vi "Update Core.vi"(8 "error in (no error)":cluster{"状态":bool, "代码":i32, "源":string} caption="错误输入（无错误）", 11 "水位控制器输入":refnum<class "Level Controller.lvclass">) -> (0 "error out":cluster{"状态":bool, "代码":i32, "源":string} caption="错误输出", 3 "水位控制器输出":refnum<class "Level Controller.lvclass">)   [LabVIEW 2015, in "Level Controller.lvlib" / "Level Controller.lvclass"]
doc: "子类绝不可对该VI进行重写。该VI通过“定时循环操作者”父类定义。该水位控制器中，“更新”操作即对水位控制器监控的变量进行检查，然后根据该变量是否高于/低于死区范围执行状态更改。"
uses:
  Level Controller.lvclass
  Level Controller.lvclass/Level Controller.ctl
  Value Position.ctl
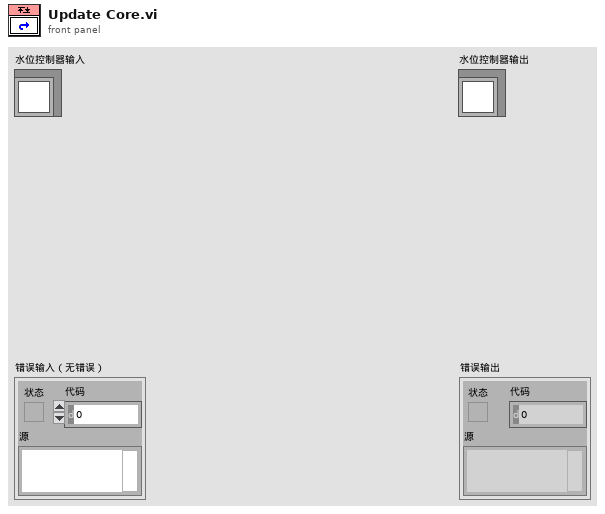
[diagram p1: front panel]
types:
  T1 = typedef "Level Controller.lvlib/Level Controller.lvclass/Value Position.ctl" = enum16{"Never Assigned", "Above Level", "Below Level"}
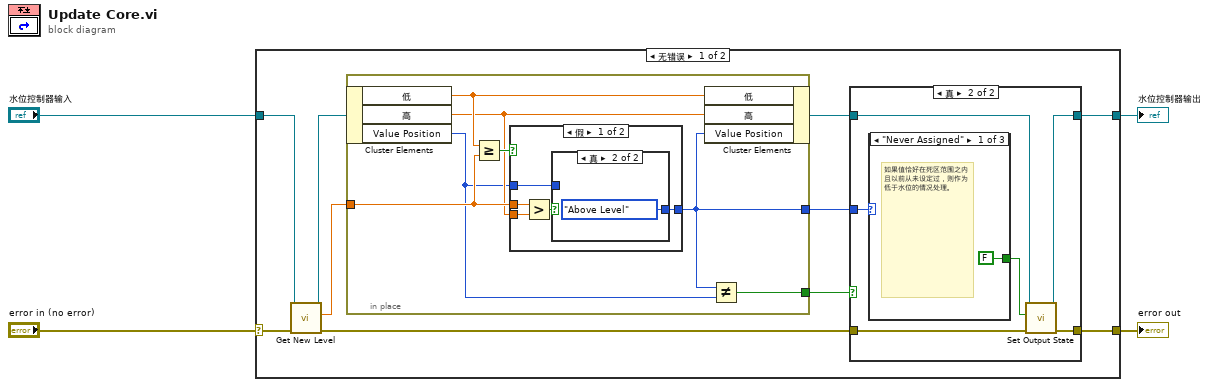
[diagram p0: block diagram]
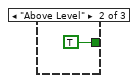
[diagram p3: hidden frame]
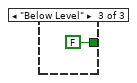
[diagram p4: hidden frame]
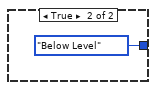
[diagram p6: hidden frame]
diagram:
  n1 = case shown="无错误" "error in (no error)" {
    selector: "error in (no error)" -> [w14 w42]
    tunnel: [w13 w42] -> w3
    tunnel: [w8 w41] -> w2
    tunnel: "水位控制器输入" -> [w10 w41]
    frame No Error {
      n2 = call-dynamic "Get New Level.vi"("error in (no error)"=w14, "水位控制器输入"=w10) -> ("error out"=w12:cluster{"状态":bool, "代码":i32, "源":string}, "水位"=w11:dbl, "水位控制器输出"=w5:refnum<class "Level Controller.lvclass">)  [unwired: 7 in]
      n3 = in-place {
        in-place-border: w11 -> [w30]
        in-place-border: [w32] -> w7
        in-place-border: [w27] -> w6
        n4 = in-place-cluster #1(w5) -> ("低"=w31:dbl, "高"=w28:dbl, "Value Position"=w26:T1)
        n5 = Greater Or Equal?(x=w31, y=w30) -> (x >= y?=w29:bool)
        n6 = case shown="假" w29 {
          tunnel: w30 -> [w37 _]
          tunnel: [w35 Value_Position."Below Level" ("Value Position")] -> w27
          tunnel: w28 -> [w36 _]
          tunnel: w26 -> [w33 _]
          frame False {
            n7 = Greater?(x=w37, y=w36) -> (0:w34:bool)
            n8 = case shown="真" w34 {
              tunnel: [w38 Value_Position."Above Level" ("Value Position")] -> w35
              tunnel: w33 -> [w38 _]
              frame False {
              }
              frame True {
              }
            }
          }
          frame True {
          }
        }
        n9 = in-place-cluster #1("低"=w31, "高"=w28, "Value Position"=w27) -> (w9:refnum<class "Level Controller.lvclass">)
        n10 = Not Equal?(x=w27, y=w26) -> (x != y?=w32:bool)
      }
      n11 = case shown="真" w7 {
        tunnel: [w15 w22] -> w13
        tunnel: w12 -> [w15 w21]
        tunnel: w9 -> [w16 w20]
        tunnel: [w16 w19] -> w8
        tunnel: w6 -> [_ w18]
        frame False {
        }
        frame True {
          n12 = case shown="\"Never Assigned\"" w18 {
            tunnel: [FALSE TRUE FALSE] -> w17
            frame "Never Assigned" {
              # "如果值恰好在死区范围之内且以前从未设定过，则作为低于水位的情况处理。"
            }
            frame "Above Level" {
            }
            frame "Below Level" {
            }
          }
          n13 = call-dynamic "Set Output State.vi"("error in (no error)"=w21, "输出状态"=w17, "水位控制器输入"=w20) -> ("error out"=w22:cluster{"状态":bool, "代码":i32, "源":string}, "水位控制器输出"=w19:refnum<class "Level Controller.lvclass">)  [unwired: 7 in]
        }
      }
    }
    frame Error {
    }
  }
  "error out" <- w3
  "水位控制器输出" <- w2
